vi "Polling.vi"() -> ()   [LabVIEW 2018]
uses:
  <vilib>/Utility/miscctls.llb/LVPoint32TypeDef.ctl
panel:
  out "좌표":T1
  out "현재 시간":timestamp
  in  "시간 확인":bool
  out "반복":i32
  in  "정지":bool
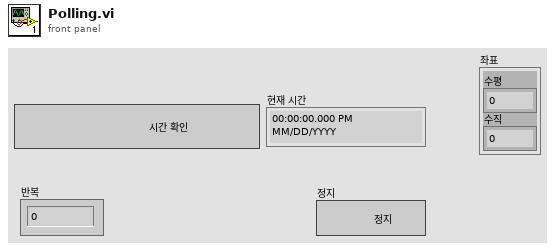
[diagram p1: front panel]
types:
  T1 = typedef "LVPoint32TypeDef.ctl" = cluster{"Horizontal":i32, "Vertical":i32}
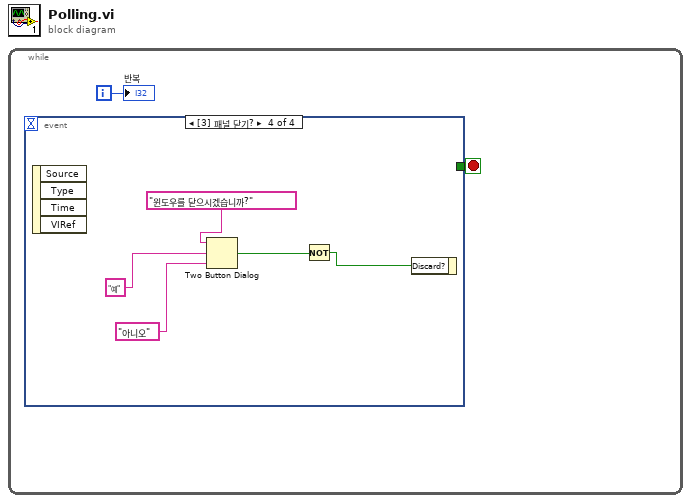
[diagram p0: block diagram]
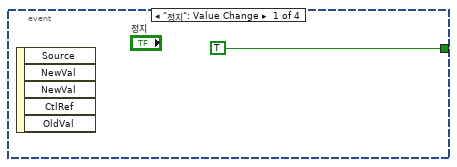
[diagram p2: hidden frame]
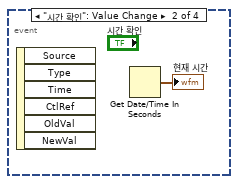
[diagram p3: hidden frame]
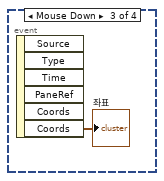
[diagram p4: hidden frame]
diagram:
  n1 = while {
    i -> [w2]
    stop <- w1 stop-if-true
    n2 = event shown="[3] 패널 닫기?" {
      selector: _ -> [_ _ _ _]
      dyn-events: _ -> [_ _ _ _]
      timeout: _ -> [_ _ _ _]
      tunnel: [TRUE _ _ _] -> w1
      event "정지": Value Change {
        n3 = event-data() -> ()  [unwired: 1 in, 5 out]
      }
      event "시간 확인": Value Change {
        n4 = event-data() -> ()  [unwired: 1 in, 6 out]
        n5 = Get Date/Time In Seconds() -> (seconds since 1Jan1904=→"현재 시간":timestamp)
      }
      event Mouse Down {
        n6 = event-data() -> ("Coords"=→"좌표":T1)  [unwired: 1 in, 5 out]
      }
      event Panel Close? {
        n7 = event-data() -> ()  [unwired: 1 in, 4 out]
        n8 = Two Button Dialog(message="윈도우를 닫으시겠습니까?", 1:"아니오", 2:"예") -> (T button?=w10:bool)
        n9 = Not(x=w10) -> (.not. x?=w9:bool)
        n10 = event-data("Discard?"=w9) -> ()  [unwired: 1 in, 1 out]
      }
    }
    "반복" <- w2
  }
